vi "Create_User_Event_Experiment.vi"(3 "error in (no error)":errorcluster) -> (0 "error out":errorcluster, 2 "Button_User_Event":refnum<user-event>)   [LabVIEW 2023]
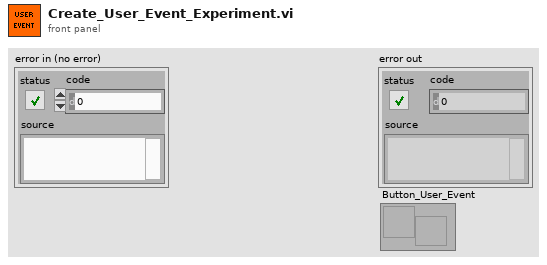
[diagram p1: front panel]
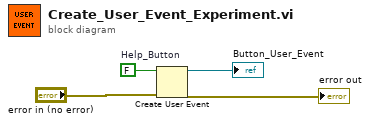
[diagram p0: block diagram]
diagram:
  w2 = FALSE  # Help_Button
  n1 = Create User Event(user event datatype=w2, error in="error in (no error)") -> (user event=→"Button_User_Event":refnum<user-event>, error out=→"error out":errorcluster)
